vi "randperm.vi"(1 "N":i32) -> (0 "permutations":i32[](array[numeric]))   [LabVIEW 2020]
doc: "Equivalent of Matlab randperm(N)."
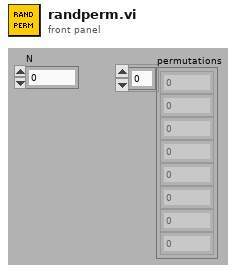
[diagram p1: front panel]
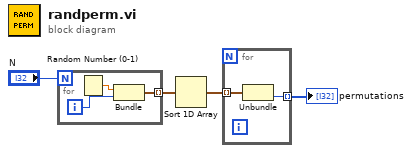
[diagram p0: block diagram]
diagram:
  n1 = for {
    N: "N" -> [_]
    tunnel: [w5] -> w3 mode=indexing
    i -> [w7]
    n2 = Random Number (0-1)() -> (number: 0 to 1=w6:dbl)
    n3 = Bundle("number: 0 to 1"=w6, w7) -> (w5:cluster{"number: 0 to 1":dbl, i32})  [unwired: 1 in]
  }
  n4 = Sort 1D Array(array=w3) -> (sorted array=w2:cluster{"number: 0 to 1":dbl, i32}[])
  n5 = for {
    tunnel: w2 -> [w9] mode=indexing
    tunnel: [w8] -> w1 mode=indexing
    n6 = Unbundle(w9) -> (w8:i32)  [unwired: 1 out]
  }
  "permutations" <- w1
